vi "Build Driver Settings Mappings.vi"(8 "error in (no error)":errorcluster, 11 "ArduinoUnoR3 in":refnum<class "ArduinoUnoR3.lvclass">) -> (0 "error out":errorcluster, 3 "ArduinoUnoR3 out":refnum<class "ArduinoUnoR3.lvclass">)   [LabVIEW 2023, in "HAF.lvlib" / "ArduinoUnoR3.lvclass"]
uses:
  ArduinoUnoR3.lvclass
  ArduinoUnoR3.lvclass/ArduinoUnoR3.ctl
  SerialDriver/SerialDriver.lvclass
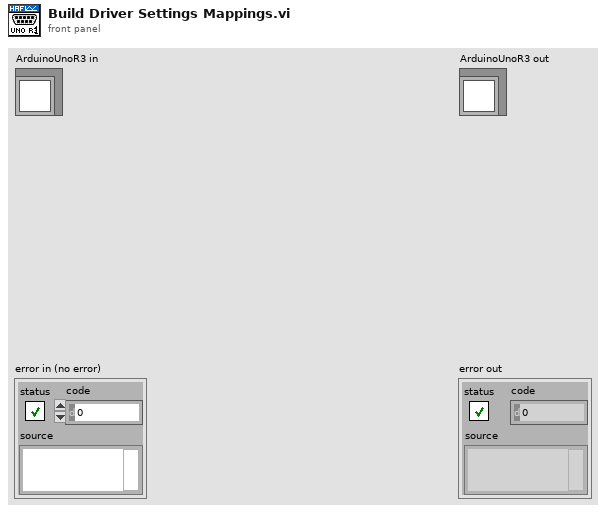
[diagram p1: front panel]
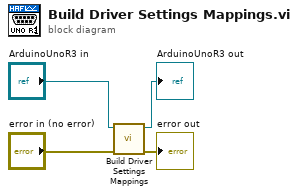
[diagram p0: block diagram]
diagram:
  n1 = call-parent "Build Driver Settings Mappings.vi"("error in (no error)"="error in (no error)", "Driver in"="ArduinoUnoR3 in") -> ("error out"=→"error out":errorcluster, "Driver out"=→"ArduinoUnoR3 out":refnum<class "ArduinoUnoR3.lvclass">)  [unwired: 8 in]
